vi "teleop_balance.vi"() -> (0 "In Range?":bool, 3 "forward power":dbl)   [LabVIEW 2020]
doc: "Calculates motor power to balance on the charging station. Returns true when within exceptable level range."
uses:
  Robot Global Data.vi
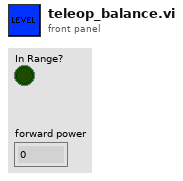
[diagram p1: front panel]
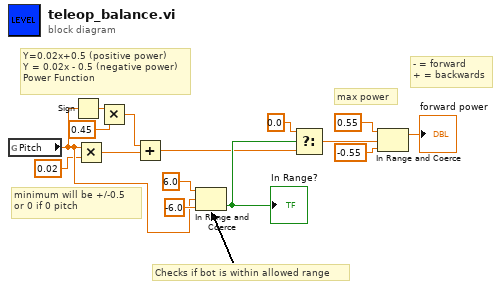
[diagram p0: block diagram]
diagram:
  # "max power"
  # "Checks if bot is within allowed range"
  # "minimum will be +/-0.5\nor 0 if 0 pitch"
  # "Y=0.02x+0.5 (positive power)\nY = 0.02x - 0.5 (negative power)\nPower Function"
  # "- = forward\n+ = backwards"
  n1 = global read "Robot Global Data.vi" "Pitch"() -> (w5:dbl)
  n2 = Sign(1:w5) -> (0:w7:dbl)
  n3 = Multiply(x=w5, y=0.02) -> (x*y=w1:dbl)
  n4 = Multiply(x=w7, y=0.45) -> (x*y=w2:dbl)
  n5 = Add(x=w2, y=w1) -> (x+y=w3:dbl)
  n6 = In Range and Coerce(upper limit=6.0, x=w5, lower limit=-6.0) -> (In Range?=w10:bool)  [unwired: 1 out]
  "In Range?" <- w10
  n7 = Select(t=0.0, s=w10, f=w3) -> (s? t:f=w8:dbl)
  n8 = In Range and Coerce(upper limit=0.55, x=w8, lower limit=-0.55) -> (coerced(x)=→"forward power":dbl)  [unwired: 1 out]
